vi "sub_strain_filter_n_offset.vi"(7 "nulling":bool, 11 "Strain raw wf":waveform(dbl)[](array[waveform])) -> (3 "strain filter_n_nulling wf":waveform(dbl)[](array[waveform]))   [LabVIEW 2016]
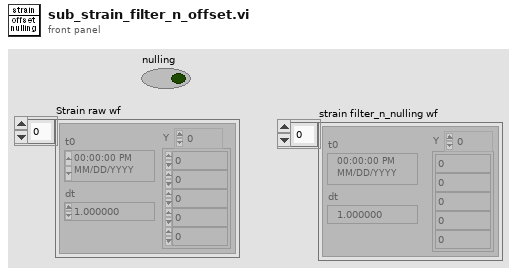
[diagram p1: front panel]
types:
  T1 = typedef "config_ctl.ctl" = cluster{"Lower Cut-Off":dbl, "Vacuum Trigger level":dbl, "state settings":cluster{"method":enum32{"histogram", "peak", "auto select"}, "histogram size":i32, "histogram method":enum16{"mode"}, "reserved":dbl}, "SPA-300 Setting":cluster{"Bonding force (g)":dbl, "Bonding time (ms)":dbl, "Pickup force (g)":dbl, "Pickup time (ms)":dbl, "Speed":enum16{"Slow", "Fast"}}, "sensor file":path}
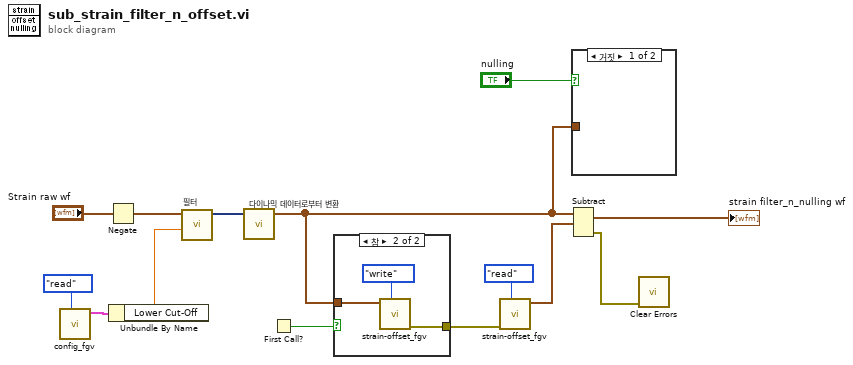
[diagram p0: block diagram]
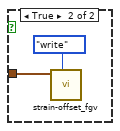
[diagram p3: hidden frame]
diagram:
  n1 = call "config_fgv.vi"("cmd"=enum16{"write", "read", "ini"}."read") -> ("Config out"=w11:T1)  [unwired: 9 in, 1 out]
  n2 = Negate(x="Strain raw wf") -> (-x=w12:waveform(dbl)[])
  n3 = Unbundle By Name(w11) -> ("Lower Cut-Off"=w8:dbl)
  n4 = call "필터"("Lower Cut-Off"=w8, "Signal"=w12) -> ("Filtered Signal"=w9:dynamicdata)  [unwired: 8 in, 1 out]
  n5 = call "다이나믹 데이터로부터 변환"("Dynamic Data Type"=w9) -> ("Array of Waveform"=w2:waveform(dbl)[])  [unwired: 3 in]
  n6 = First Call?() -> (First Call?: T/F=w3:bool)
  n7 = case shown="참" w3 {
    tunnel: [_ w16] -> w4
    tunnel: w2 -> [_ w15]
    frame False {
    }
    frame True {
      n8 = call "strain-offset_fgv.vi"("cmd"=enum16{"ini", "write", "read"}."write", "data"=w15) -> ("error out"=w16:errorcluster)  [unwired: 8 in, 1 out]
    }
  }
  n9 = call "strain-offset_fgv.vi"("cmd"=enum16{"ini", "write", "read"}."read", "error in (no error)"=w4) -> ("Strain_offset_data"=w6:waveform(dbl)[])  [unwired: 8 in, 1 out]
  n10 = Subtract(1:w6, 2:w2) -> (0:→"strain filter_n_nulling wf":waveform(dbl)[], 3:w1:errorcluster)  [unwired: 1 in]
  n11 = case shown="거짓" "nulling" {
    tunnel: w2 -> [_ w18]
    frame False {
    }
    frame True {
      n12 = call "strain-offset_fgv.vi"("cmd"=enum16{"ini", "write", "read"}."write", "data"=w18) -> ()  [unwired: 8 in, 2 out]
    }
  }
  n13 = call <vilib>:"Clear Errors.vi"("error in (no error)"=w1) -> ()  [unwired: 5 in, 2 out]
